vi "destroy.vi"(8 "error in":errorcluster, 11 "identifying queue reporter in":refnum<class "identifying queue reporter.lvclass">) -> (0 "error out":errorcluster)   [LabVIEW 2015, in "identifying queue reporter.lvclass"]
uses:
  identifying queue reporter.lvclass
  identifying queue reporter.lvclass/identifying queue reporter.ctl
  communicator queue/identifying queue.lvclass
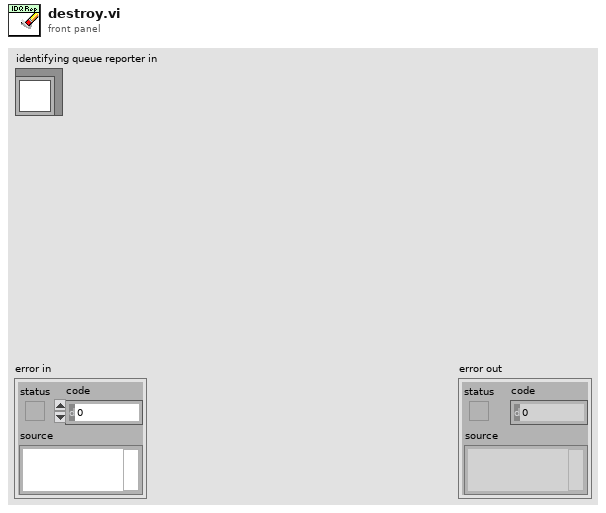
[diagram p1: front panel]
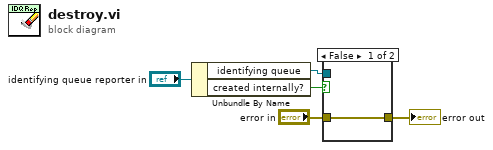
[diagram p0: block diagram]
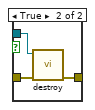
[diagram p2: hidden frame]
diagram:
  n1 = Unbundle By Name("identifying queue reporter in") -> ("identifying queue"=w3:refnum<class "identifying queue.lvclass">, "created internally?"=w2:bool)
  n2 = case shown="False" w2 {
    tunnel: "error in" -> [w6 w9]
    tunnel: w3 -> [_ w8]
    tunnel: [w6 w7] -> w1
    frame False {
    }
    frame True {
      n3 = call "destroy.vi"("error in"=w9, "message connection in"=w8) -> ("error out"=w7:errorcluster)  [unwired: 9 in]
    }
  }
  "error out" <- w1
